vi "Has Error.vi"(8 "error in (no error)":errorcluster, 11 "Listener Command in":T1=enum."Open") -> (0 "error out":errorcluster, 3 "Listener Command out":T1=enum."Open")   [LabVIEW 2019, in "Listener.lvlib"]
uses:
  Listener.lvlib
  Listener Command.ctl
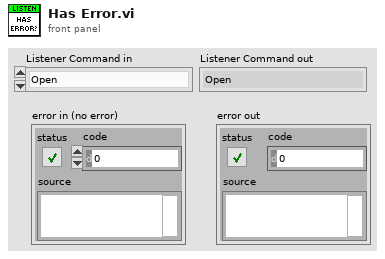
[diagram p1: front panel]
types:
  T1 = typedef "Listener.lvlib/Listener Command.ctl" = enum16{"Idle", "Open", "Incoming", "Close", "Error", "Stop"}
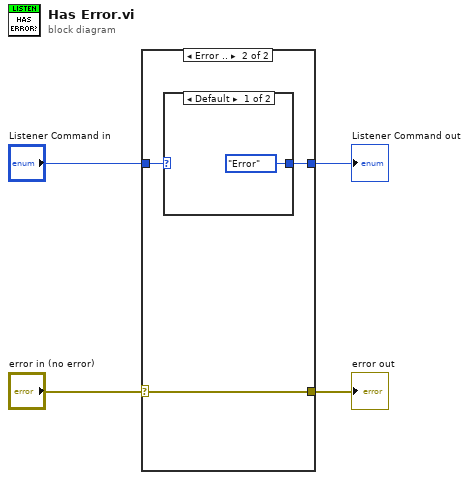
[diagram p0: block diagram]
diagram:
  n1 = case shown="Error .." "error in (no error)" {
    selector: "error in (no error)" -> [w6 w9]
    tunnel: [w6 w9] -> w3
    tunnel: [w5 w7] -> w2
    tunnel: "Listener Command in" -> [w5 w8]
    frame No Error {
    }
    frame Error {
      n2 = case shown="Default" w8 {
        selector: w8 -> [_ w11]
        tunnel: [Listener_Command."Error" ("MDS Command in") w11] -> w7
        frame Default {
        }
        frame "Stop" {
          # "already handled"
        }
      }
    }
  }
  "error out" <- w3
  "Listener Command out" <- w2
